vi "MAV_CMD_DO_SET_SERVO.vi"(9 "PWM (1000 to 2000)":sgl, 10 "Servo Number":sgl, 11 "Target System and Target Component":u8=1) -> (3 "MAVLink Message":u8[](array[numeric]))   [LabVIEW 2014]
panel:
  out "Payload Size":i32
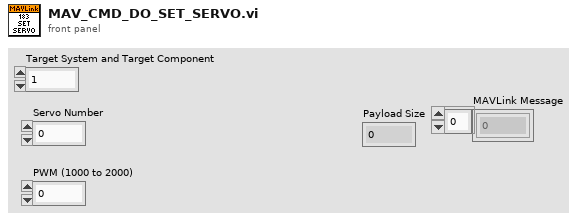
[diagram p1: front panel]
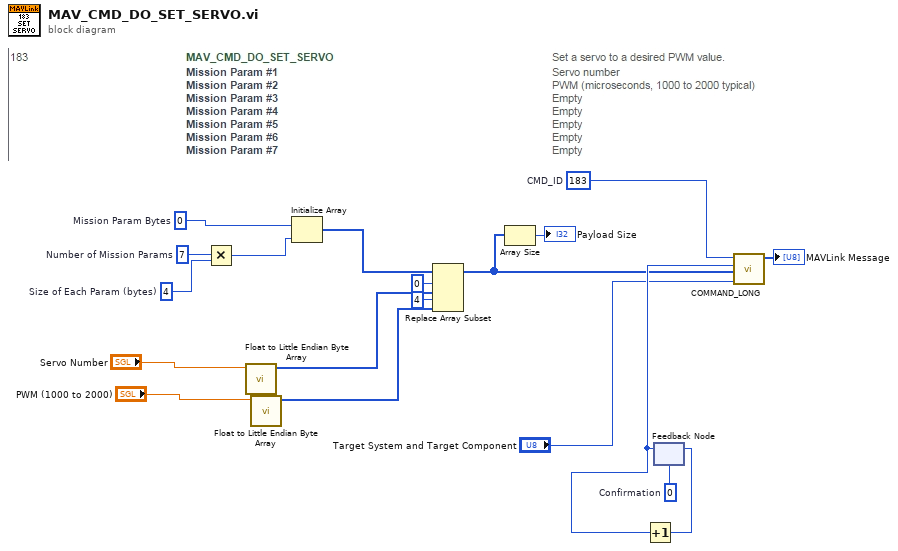
[diagram p0: block diagram]
diagram:
  w12 = u8 0  # Confirmation
  w17 = 4  # Size of Each Param (bytes)
  w18 = 7  # Number of Mission Params
  w19 = u8 0  # Mission Param Bytes
  w8 = u16 183  # CMD_ID
  n1 = Multiply(x=w18, y=w17) -> (x*y=w16:i32)
  n2 = call "Float to Little Endian Byte Array.vi"("Float In"="Servo Number") -> ("LE Byte Array"=w9:u8[])  [unwired: 10 in]
  n3 = call "Float to Little Endian Byte Array.vi"("Float In"="PWM (1000 to 2000)") -> ("LE Byte Array"=w2:u8[])  [unwired: 10 in]
  n4 = Initialize Array(w19, w16) -> (w15:u8[])
  n5 = Replace Array Subset(array=w15, new element #1=w9, index #1=0 ("index"), new element #2=w2, index #2=4 ("index")) -> (w6:u8[])
  n6 = Array Size(array=w6) -> (size(s)=→"Payload Size":i32)
  n7 = feedback #1(w12) -> (w7:u8)
  n8 = Increment(x=w7) -> (x+1=w11:u8)
  n9 = feedback-in #1(w11) -> ()
  n10 = call "COMMAND_LONG.vi"("Target System and Target Component"="Target System and Target Component", "Mission Params"=w6, "Confirmation"=w7, "Command ID"=w8) -> ("MAVLink Message"=→"MAVLink Message":u8[])  [unwired: 7 in]
